vi "Create Events.vi"(0 "Display State In":T2, 9 "Container State":T5, 11 "error in (no error)":errorcluster) -> (4 "Display State Out":T2, 8 "Events":T1, 15 "error out":errorcluster)   [LabVIEW 2015, in "SignalManager.xctl"]
uses:
  SignalManager.xctl
  <vilib>/_xctls/Container State.ctl
  State.ctl
  Utility VIs/Controls/KListboxEx/Events.ctl
  Utility VIs/Controls/KListboxEx/Event Action.ctl
  PeriodDisplay.ctl
  Events.ctl
  Event Data.ctl
  <vilib>/_xctls/XControlSupport.lvlib
  Utility VIs/Controls/KListboxEx/KListboxEx.xctl
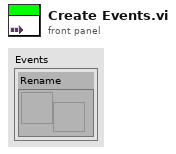
[diagram p1: front panel]
types:
  T1 = typedef "SignalManager.xctl/Events.ctl" = cluster{"Rename":refnum<user-event>}
  T2 = typedef "SignalManager.xctl/State.ctl" = cluster{"Channels":T3, "Destinations":string[], "action":string, "EventReg":refnum<event-registration>, "selectedChan":i32, "Period Display":T4, "Events":T1}
  T3 = typedef "KListboxEx.xctl/Events.ctl" = cluster{"Items Changed":refnum<user-event>, "List Changed":refnum<user-event>}
  T4 = typedef "SignalManager.xctl/PeriodDisplay.ctl" = enum16{"Interval", "RepRate", "Both"}
  T5 = typedef "XControlSupport.lvlib/Container State.ctl" = cluster{"Indicator?":bool, "Run Mode?":bool, " Refnum":refnum<vi>}
  T6 = typedef "SignalManager.xctl/Event Data.ctl" = cluster{"Old name":string, "New name":string}
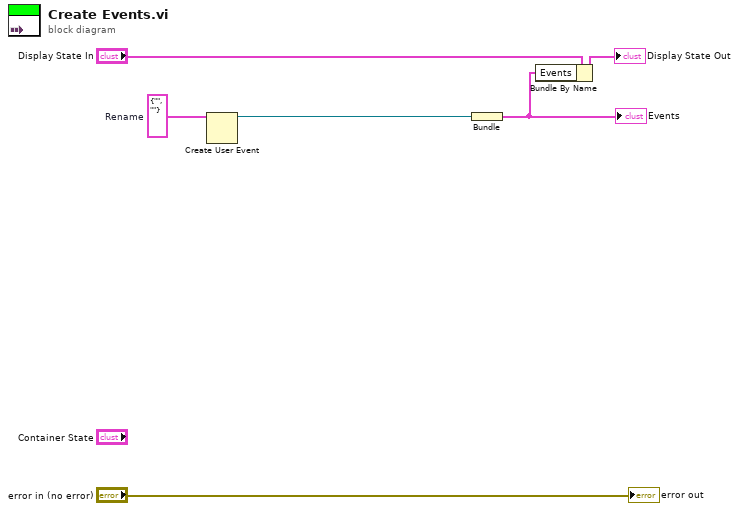
[diagram p0: block diagram]
diagram:
  w4 = T6 {"Old name"="", "New name"=""}  # Rename
  n1 = Create User Event(user event datatype=w4) -> (user event=w2:refnum<user-event>)  [unwired: 1 in, 1 out]
  n2 = Bundle("Rename"=w2) -> (w1:cluster{"Rename":refnum<user-event>})  [unwired: 1 in]
  "Events" <- w1
  n3 = Bundle By Name(cluster="Display State In", "Events"=w1) -> (→"Display State Out":T2)
  "error out" <- "error in (no error)"
